vi "LV_UNIXTIME.vi"(11 "current time":timestamp) -> (0 "date/time string":string, 2 "UNIX time (s)":dbl format="%#_13f")   [LabVIEW 2017]
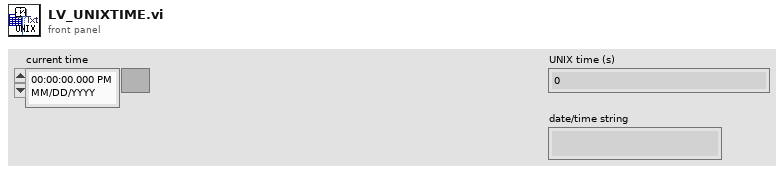
[diagram p1: front panel]
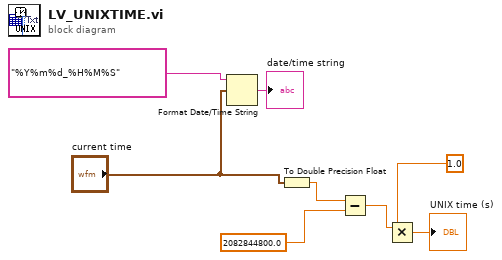
[diagram p0: block diagram]
diagram:
  n1 = Format Date/Time String(time format string (%c)="%Y%m%d_%H%M%S", seconds (now)="current time") -> (date/time string=→"date/time string":string)  [unwired: 1 in]
  n2 = To Double Precision Float(number="current time") -> (double precision float=w8:dbl)
  n3 = Subtract(x=w8, y=2082844800.0) -> (x-y=w6:dbl)
  n4 = Multiply(x=w6, y=1.0) -> (x*y=→"UNIX time (s)":dbl)
